vi "sv_Get HV Weighting Filter Coefficients.vi"(6 "reset filter (F)":bool, 8 "error in (no error)":errorcluster, 9 "weighting filter":T2 items=["Linear", "A-weighting", "B-weighting", "C-weighting", "ITU-R 468-4", "Dolby", "CCITT", "C-message", "Wb", "Wc", "Wd", "We", "Wf", "Wh", "Wj", "Wk", "Wm", "AES17 20 kHz lowpass", "AES17 40 kHz lowpass", "AES17 20 kHz highpass", "AES17 40 kHz highpass"], 11 "scaled signal":waveform(dbl)={"t0"=timestamp(0 s since 1904-01-01), "dt"=0.0, "Y"=[]}) -> (0 "error out":errorcluster, 1 "a-v filter coefficients":T1 {"Forward Coefficients" format="%.4f"; "Reverse Coefficients" format="%.4f"}, 2 "LP filter coefficients":T1 {"Forward Coefficients" format="%.4f"; "Reverse Coefficients" format="%.4f"}, 3 "dup scaled signal":waveform(dbl), 4 "upward step filter coefficients":T1 {"Forward Coefficients" format="%.4f"; "Reverse Coefficients" format="%.4f"}, 5 "HP filter coefficients":T1 {"Forward Coefficients" format="%.4f"; "Reverse Coefficients" format="%.4f"})   [LabVIEW 2017]
doc: "Designs the A, B, or C weighting filter coefficients. The design is based on the ANSI S1.42-1986 standard. This VI also returns the maximum frequency, expressed in hertz, within the tolerance limits based on the selected type (Type 1 or Type 0), according to the ANSI S1.4-1986 standard."
uses:
  <vilib>/addons/_NISVFA/_Shared subVIs/Controls/svc_Weighting Filter Text Ring.ctl
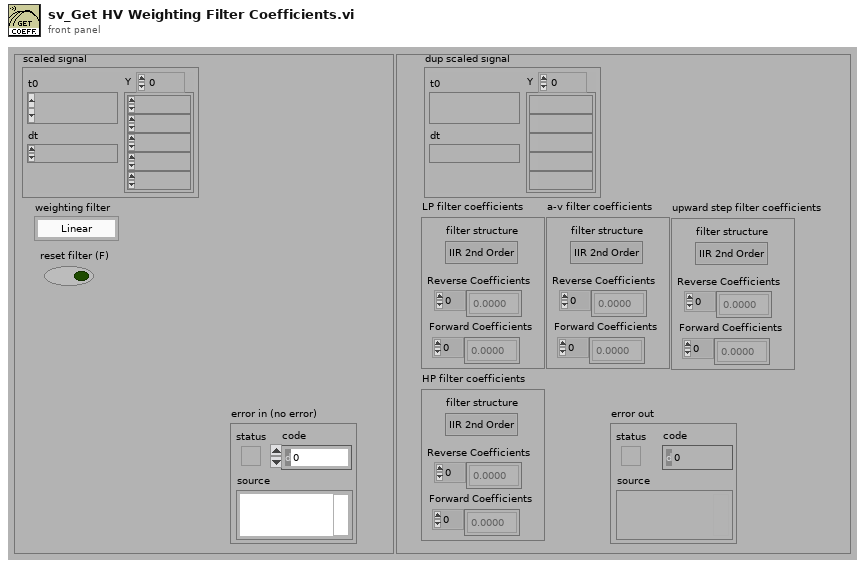
[diagram p1: front panel]
types:
  T1 = cluster{"filter structure":enum32{"IIR 2nd Order", "IIR 4th Order"}, "Reverse Coefficients":dbl[], "Forward Coefficients":dbl[]}
  T2 = typedef "svc_Weighting Filter Text Ring.ctl" = u16
  T3 = cluster{"filter structure":enum32{"IIR 2nd Order", "IIR 4th Order"}, "Reverse Coefficients":dbl[], "Forward Coefficients":dbl[]}[]
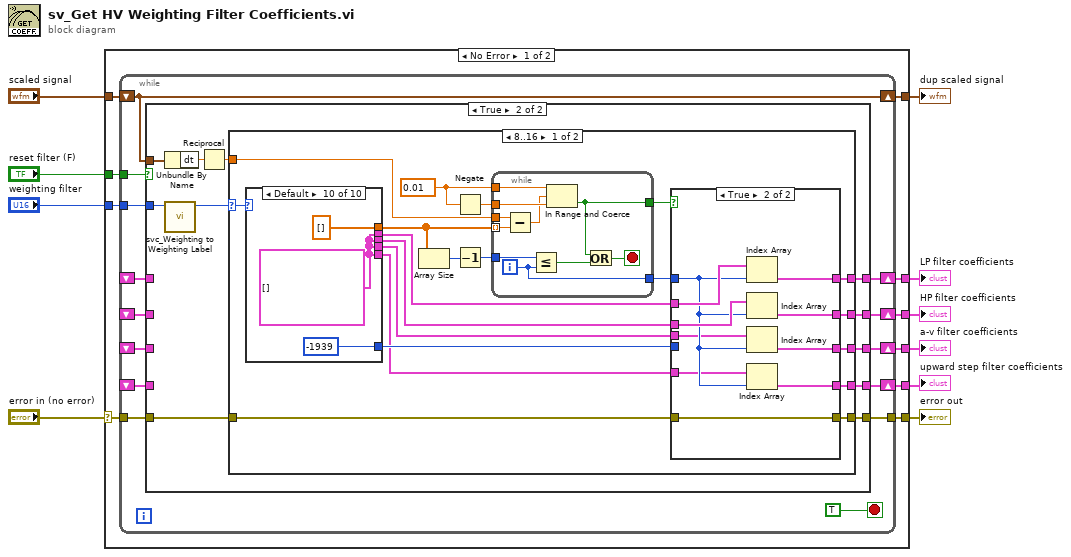
[diagram p0: block diagram]
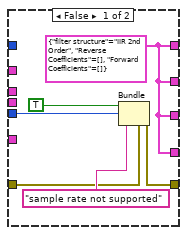
[diagram p3: hidden frame]
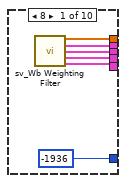
[diagram p4: hidden frame]
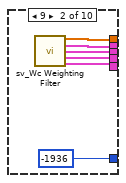
[diagram p5: hidden frame]
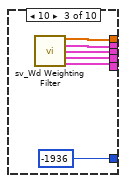
[diagram p6: hidden frame]
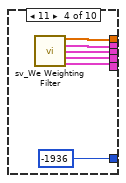
[diagram p7: hidden frame]
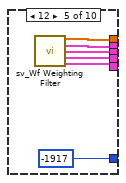
[diagram p8: hidden frame]
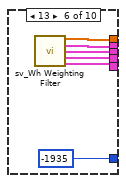
[diagram p9: hidden frame]
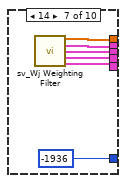
[diagram p10: hidden frame]
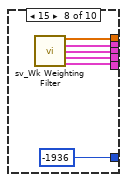
[diagram p11: hidden frame]
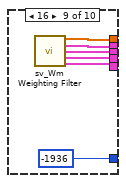
[diagram p12: hidden frame]
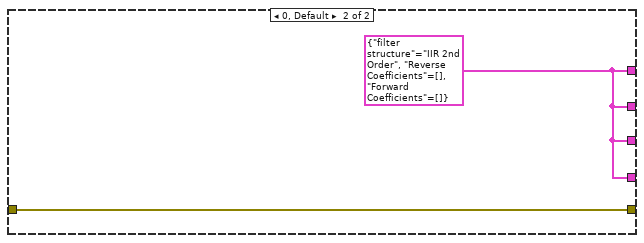
[diagram p13: hidden frame]
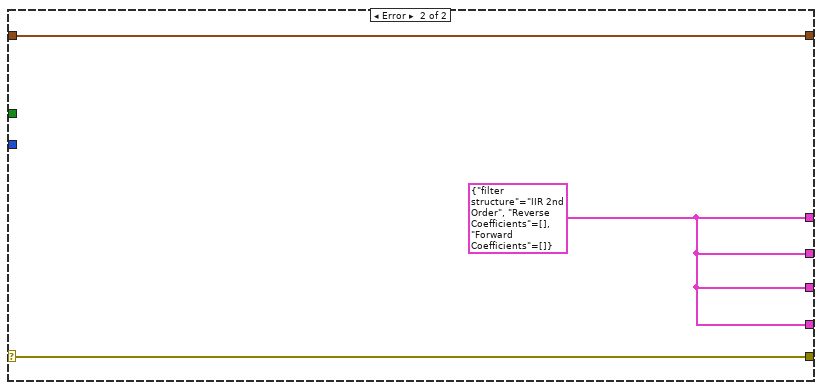
[diagram p14: hidden frame]
diagram:
  n1 = case shown="No Error" "error in (no error)" {
    selector: "error in (no error)" -> [w15 w158]
    tunnel: [w20 w156] -> w10
    tunnel: "scaled signal" -> [w18 w157]
    tunnel: [w14 w158] -> w8
    tunnel: [w17 w157] -> w6
    tunnel: "weighting filter" -> [w19 _]
    tunnel: "reset filter (F)" -> [w16 _]
    tunnel: [w13 w156] -> w3
    tunnel: [w12 w156] -> w2
    tunnel: [w11 w156] -> w1
    frame No Error {
      n2 = while {
        tunnel: w19 -> [w33]
        tunnel: w16 -> [w30]
        shift-right: [w34] -> w20
        shift-left: _ -> [w29]
        tunnel: w15 -> [w28]
        tunnel: [w27] -> w14
        shift-right: [w31] -> w17
        shift-left: w18 -> [w31]
        shift-right: [w26] -> w13
        shift-left: _ -> [w23]
        shift-right: [w25] -> w12
        shift-left: _ -> [w22]
        shift-right: [w24] -> w11
        shift-left: _ -> [w21]
        stop <- TRUE stop-if-true
        n3 = case shown="True" w30 {
          tunnel: [w39 w50] -> w34
          tunnel: w33 -> [_ w46]
          tunnel: w31 -> [_ w45]
          tunnel: w29 -> [w39 _]
          tunnel: w28 -> [w38 w44]
          tunnel: [w38 w43] -> w27
          tunnel: [w37 w42] -> w26
          tunnel: [w36 w41] -> w25
          tunnel: [w35 w40] -> w24
          tunnel: w23 -> [w37 _]
          tunnel: w22 -> [w36 _]
          tunnel: w21 -> [w35 _]
          frame False {
          }
          frame True {
            n4 = Unbundle By Name(w45) -> ("dt"=w49:dbl)
            n5 = call <vilib>:"svc_Weighting to Weighting Label.vi"("weighting filter"=w46) -> ("weighting enum"=w47:T2)  [unwired: 9 in, 1 out]
            n6 = Reciprocal(x=w49) -> (1/x=w48:dbl)
            n7 = case shown="8..16" w47 {
              selector: w47 -> [w70 _]
              tunnel: [w63 w154] -> w50
              tunnel: w48 -> [w67 _]
              tunnel: w44 -> [w62 w155]
              tunnel: [w61 w155] -> w43
              tunnel: [w53 w154] -> w42
              tunnel: [w52 w154] -> w41
              tunnel: [w51 w154] -> w40
              frame 8..16 {
                w57 = 0.01
                n8 = case shown="Default" w70 {
                  tunnel: [w102 w108 w114 w120 w126 w132 w138 w144 w150 dbl[] []] -> w60
                  tunnel: [w101 w107 w113 w119 w125 w131 w137 w143 w149 w151] -> w59
                  tunnel: [-1936 ("code") -1936 ("code") -1936 ("code") -1936 ("code") -1917 ("code") -1935 ("code") -1936 ("code") -1936 ("code") -1936 ("code") -1939 ("code")] -> w58
                  tunnel: [w99 w105 w111 w117 w123 w129 w135 w141 w147 w151] -> w56
                  tunnel: [w98 w104 w110 w116 w122 w128 w134 w140 w146 w151] -> w55
                  tunnel: [w97 w103 w109 w115 w121 w127 w133 w139 w145 w151] -> w54
                  frame 8 {
                    n9 = call <vilib>:"sv_Wb Weighting Filter.vi"() -> ("supported sample rates"=w102:dbl[], "low pass time-domain Wb filters at supported sampe rates"=w101:T3, "high pass time-domain Wb filters at supported sampe rates"=w99:T3, "a-v time-domain Wb filters at supported sampe rates"=w98:T3, "upward step time-domain Wb filters at supported sampe rates"=w97:T3)  [unwired: 11 in]
                  }
                  frame 9 {
                    n10 = call <vilib>:"sv_Wc Weighting Filter.vi"() -> ("supported sample rates"=w108:dbl[], "low pass time-domain Wc filters at supported sampe rates"=w107:T3, "high pass time-domain Wc filters at supported sampe rates"=w105:T3, "a-v time-domain Wc filters at supported sampe rates"=w104:T3, "upward step time-domain Wc filters at supported sampe rates"=w103:T3)  [unwired: 11 in]
                  }
                  frame 10 {
                    n11 = call <vilib>:"sv_Wd Weighting Filter.vi"() -> ("supported sample rates"=w114:dbl[], "low pass time-domain Wd filters at supported sampe rates"=w113:T3, "high pass time-domain Wd filters at supported sampe rates"=w111:T3, "a-v time-domain Wd filters at supported sampe rates"=w110:T3, "upward step time-domain Wd filters at supported sampe rates"=w109:T3)  [unwired: 11 in]
                  }
                  frame 11 {
                    n12 = call <vilib>:"sv_We Weighting Filter.vi"() -> ("supported sample rates"=w120:dbl[], "low pass time-domain Wd filters at supported sampe rates"=w119:T3, "high pass time-domain Wd filters at supported sampe rates"=w117:T3, "a-v time-domain Wd filters at supported sampe rates"=w116:T3, "upward step time-domain Wd filters at supported sampe rates"=w115:T3)  [unwired: 11 in]
                  }
                  frame 12 {
                    n13 = call <vilib>:"sv_Wf Weighting Filter.vi"() -> ("supported sample rates"=w126:dbl[], "low pass time-domain Wf filters at supported sampe rates"=w125:T3, "high pass time-domain Wf filters at supported sampe rates"=w123:T3, "a-v time-domain Wf filters at supported sampe rates"=w122:T3, "upward step time-domain Wf filters at supported sampe rates"=w121:T3)  [unwired: 11 in]
                  }
                  frame 13 {
                    n14 = call <vilib>:"sv_Wh Weighting Filter.vi"() -> ("supported sample rates"=w132:dbl[], "low pass time-domain Wh filters at supported sampe rates"=w131:T3, "high pass time-domain Wh filters at supported sampe rates"=w129:T3, "a-v time-domain Wh filters at supported sampe rates"=w128:T3, "upward step time-domain Wh filters at supported sampe rates"=w127:T3)  [unwired: 11 in]
                  }
                  frame 14 {
                    n15 = call <vilib>:"sv_Wj Weighting Filter.vi"() -> ("supported sample rates"=w138:dbl[], "low pass time-domain Wh filters at supported sampe rates"=w137:T3, "high pass time-domain Wh filters at supported sampe rates"=w135:T3, "a-v time-domain Wh filters at supported sampe rates"=w134:T3, "upward step time-domain Wh filters at supported sampe rates"=w133:T3)  [unwired: 11 in]
                  }
                  frame 15 {
                    n16 = call <vilib>:"sv_Wk Weighting Filter.vi"() -> ("supported sample rates"=w144:dbl[], "low pass time-domain Wh filters at supported sampe rates"=w143:T3, "high pass time-domain Wh filters at supported sampe rates"=w141:T3, "a-v time-domain Wh filters at supported sampe rates"=w140:T3, "upward step time-domain Wh filters at supported sampe rates"=w139:T3)  [unwired: 11 in]
                  }
                  frame 16 {
                    n17 = call <vilib>:"sv_Wm Weighting Filter.vi"() -> ("supported sample rates"=w150:dbl[], "low pass time-domain Wh filters at supported sampe rates"=w149:T3, "high pass time-domain Wh filters at supported sampe rates"=w147:T3, "a-v time-domain Wh filters at supported sampe rates"=w146:T3, "upward step time-domain Wh filters at supported sampe rates"=w145:T3)  [unwired: 11 in]
                  }
                  frame Default {
                    w151 = T3 []
                  }
                }
                n18 = Array Size(array=w60) -> (size(s)=w69:i32)
                n19 = Negate(x=w57) -> (-x=w66:dbl)
                n20 = Decrement(x=w69) -> (x-1=w68:i32)
                n21 = while {
                  tunnel: w68 -> [w93]
                  tunnel: w67 -> [w96]
                  tunnel: w60 -> [w95] mode=indexing
                  tunnel: w57 -> [w90]
                  tunnel: w66 -> [w89]
                  tunnel: [w91] -> w64
                  tunnel: [w88] -> w65
                  i -> [w91]
                  stop <- w94 stop-if-true
                  n22 = Subtract(x=w96, y=w95) -> (x-y=w87:dbl)
                  n23 = Less Or Equal?(x=w93, y=w91) -> (x <= y?=w92:bool)
                  n24 = In Range and Coerce(upper limit=w90, x=w87, lower limit=w89) -> (In Range?=w88:bool)  [unwired: 1 out]
                  n25 = Or(x=w88, y=w92) -> (x .or. y?=w94:bool)
                }
                n26 = case shown="True" w65 {
                  tunnel: w59 -> [_ w86]
                  tunnel: w64 -> [_ w82]
                  tunnel: [w71 w85] -> w63
                  tunnel: w62 -> [w73 w84]
                  tunnel: [w74 w84] -> w61
                  tunnel: w58 -> [w76 _]
                  tunnel: w56 -> [_ w83]
                  tunnel: w55 -> [_ w81]
                  tunnel: w54 -> [_ w80]
                  tunnel: [w71 w79] -> w53
                  tunnel: [w71 w78] -> w52
                  tunnel: [w71 w77] -> w51
                  frame False {
                    w71 = T1 {"filter structure"=enum."IIR 2nd Order", "Reverse Coefficients"=[], "Forward Coefficients"=[]} ("filter coefficients")
                    n27 = Bundle(cluster=w73, "status"=TRUE, "code"=w76, "source"="sample rate not supported") -> (w74:errorcluster)
                  }
                  frame True {
                    n28 = Index Array(array=w86, index=w82) -> (element=w85:T1)
                    n29 = Index Array(array=w83, index=w82) -> (element=w79:T1)
                    n30 = Index Array(array=w81, index=w82) -> (element=w78:T1)
                    n31 = Index Array(array=w80, index=w82) -> (element=w77:T1)
                  }
                }
              }
              frame 0, Default {
                w154 = T1 {"filter structure"=enum."IIR 2nd Order", "Reverse Coefficients"=[], "Forward Coefficients"=[]} ("filter coefficients")
              }
            }
          }
        }
      }
    }
    frame Error {
      w156 = T1 {"filter structure"=enum."IIR 2nd Order", "Reverse Coefficients"=[], "Forward Coefficients"=[]} ("filter coefficients")
    }
  }
  "LP filter coefficients" <- w10
  "dup scaled signal" <- w6
  "error out" <- w8
  "HP filter coefficients" <- w3
  "a-v filter coefficients" <- w2
  "upward step filter coefficients" <- w1
